vi "LVITX append letter to filename.vi"(1 "string in":string) -> (0 "string out":string)   [LabVIEW 2011]
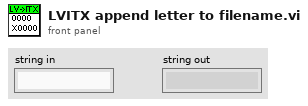
[diagram p1: front panel]
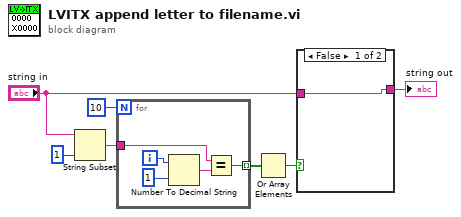
[diagram p0: block diagram]
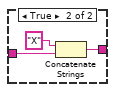
[diagram p2: hidden frame]
diagram:
  n1 = String Subset(string="string in", length (rest)=1 ("length (rest)")) -> (substring=w5:string)  [unwired: 1 in]
  n2 = for {
    N: 10 -> [_]
    tunnel: w5 -> [w9]
    tunnel: [w8] -> w4 mode=indexing
    i -> [w11]
    n3 = Number To Decimal String(number=w11, width (-)=i16 1) -> (decimal integer string=w10:string)
    n4 = Equal?(x=w9, y=w10) -> (x = y?=w8:bool)
  }
  n5 = Or Array Elements(Boolean array=w4) -> (logical OR=w2:bool)
  n6 = case shown="False" w2 {
    tunnel: "string in" -> [w13 w16]
    tunnel: [w13 w14] -> w1
    frame False {
    }
    frame True {
      n7 = Concatenate Strings("X" ("string"), w16) -> (w14:string)
    }
  }
  "string out" <- w1
